vi "Multipath Channel (SubVI).vi"(2 "OFDM Frame":cdb[](array[numeric]), 3 "multipath":i32) -> (0 "ch_op":cdb[](array[numeric]), 1 "tap_gain_vec":cdb[](array[numeric]))   [LabVIEW 2015]
uses:
  <vilib>/gmath/statdist.llb/Normal Random.vi
  <vilib>/imath/engines/lvmath2/RunTimeEngine/BuiltInFunctions/length/NIMS_length(GV).vi
  <instcachedir>/0/NIMS_length(GV)_08A3D13377FD4E4B96F5795FBF3698FA.lvgen/NIMS_length(GV)_08A3D13377FD4E4B96F5795FBF3698FA_001.vi
  <vilib>/imath/engines/lvmath2/RunTimeEngine/BuiltInFunctions/convcirc/NIMS_convcirc(CV,CV,I32).vi
  <instcachedir>/0/NIMS_convcirc(CV,CV,I32)_57506B9F9B0742FA845FB309D2B33469.lvgen/NIMS_convcirc(CV,CV,I32)_57506B9F9B0742FA845FB309D2B33469_000.vi
  <vilib>/imath/engines/lvmath2/RunTimeEngine/ErrorHandling/NIMS_Error From Error Code.vi
  <vilib>/imath/engines/lvmath2/RunTimeEngine/NodeEndStatement/NIMS_NodeEndStatement_Output.vi
  <instcachedir>/0/NIMS_NodeEndStatement_Output_53EC0D466D134D7ABD903AC30B43404B.lvgen/NIMS_NodeEndStatement_Output_53EC0D466D134D7ABD903AC30B43404B_000.vi
  <vilib>/imath/engines/lvmath2/RunTimeEngine/ErrorHandling/NIMS_Finalize Error.vi
  <vilib>/gmath/NI_Gmath.lvlib
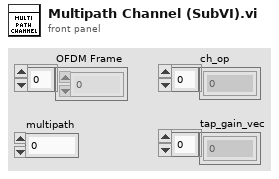
[diagram p1: front panel]
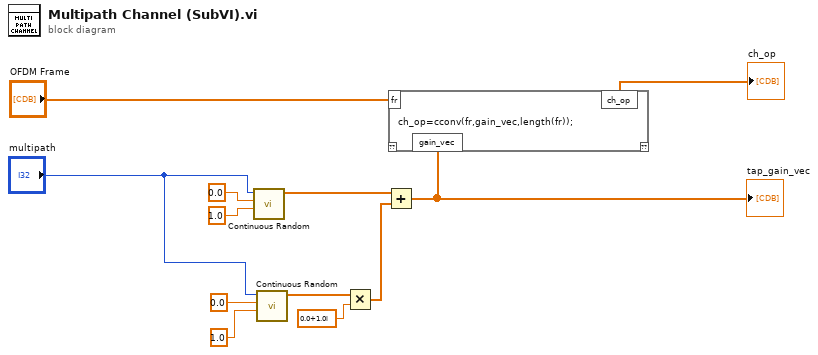
[diagram p0: block diagram]
diagram:
  n1 = call-poly <vilib>:"Continuous Random.vi"("std"=1.0, "mean"=0.0, "samples"="multipath") -> ("normal random data"=w6:dbl[])  [unwired: 7 in, 1 out]
  n2 = call-poly <vilib>:"Continuous Random.vi"("std"=1.0, "mean"=0.0, "samples"="multipath") -> ("normal random data"=w5:dbl[])  [unwired: 7 in, 1 out]
  n3 = Multiply(x=w5, y=cdb 0.0+1.0i) -> (x*y=w7:cdb[])
  n4 = Add(x=w6, y=w7) -> (x+y=w11:cdb[])
  "tap_gain_vec" <- w11
  n5 = mathscript code="ch_op=cconv(fr,gain_vec,length(fr));"("fr"="OFDM Frame", "gain_vec"=w11) -> ("ch_op"=→"ch_op":cdb[])  [unwired: 1 in, 1 out]
